vi "ma_CompleteEllipticIntegral.vi"(0 "k'":dbl=1.0 format="%0.2f") -> (1 "cei(k)":dbl format="%0.4f", 2 "convergence":bool=TRUE)   [LabVIEW 2020, in "NI_MAPro.lvlib"]
uses:
  NI_MAPro.lvlib
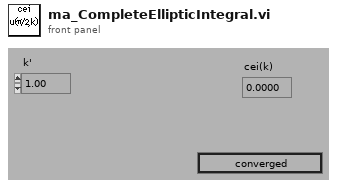
[diagram p1: front panel]
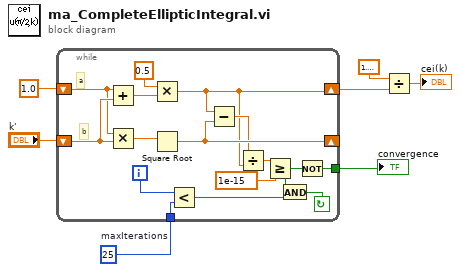
[diagram p0: block diagram]
diagram:
  w5 = 25  # maxIterations
  n1 = while {
    tunnel: [w8] -> w4
    tunnel: w5 -> [w18]
    shift-left: "k'" -> [w23]
    shift-right: [w16] -> _
    shift-left: 1.0 -> [w22]
    shift-right: [w14] -> w2
    i -> [w17]
    stop <- w9 continue-if-true
    # "b"
    # "a"
    n2 = Add(x=w22, y=w23) -> (x+y=w20:dbl)
    n3 = Multiply(x=w22, y=w23) -> (x*y=w19:dbl)
    n4 = Multiply(x=0.5, y=w20) -> (x*y=w14:dbl)
    n5 = Square Root(x=w19) -> (sqrt(x)=w16:dbl)
    n6 = Less?(x=w17, y=w18) -> (x < y?=w10:bool)
    n7 = Subtract(x=w14, y=w16) -> (x-y=w15:dbl)
    n8 = Divide(x=w15, y=w14) -> (x/y=w12:dbl)
    n9 = Greater Or Equal?(x=w12, y=1e-15) -> (x >= y?=w11:bool)
    n10 = And(x=w11, y=w10) -> (x .and. y?=w9:bool)
    n11 = Not(x=w11) -> (.not. x?=w8:bool)
  }
  "convergence" <- w4
  n12 = Divide(x=1.5707963267948966, y=w2) -> (x/y=→"cei(k)":dbl)
